vi "turn off a light.vi"(6 "error in":errorcluster, 7 "Which Button?":u32, 8 "Button 4":refnum<vi>, 9 "Button 3":refnum<vi>, 10 "Button 2":refnum<vi>, 11 "Button 1":refnum<vi>) -> (4 "error out":errorcluster)   [LabVIEW 2024]
panel:
  in  "Blank Button":bool
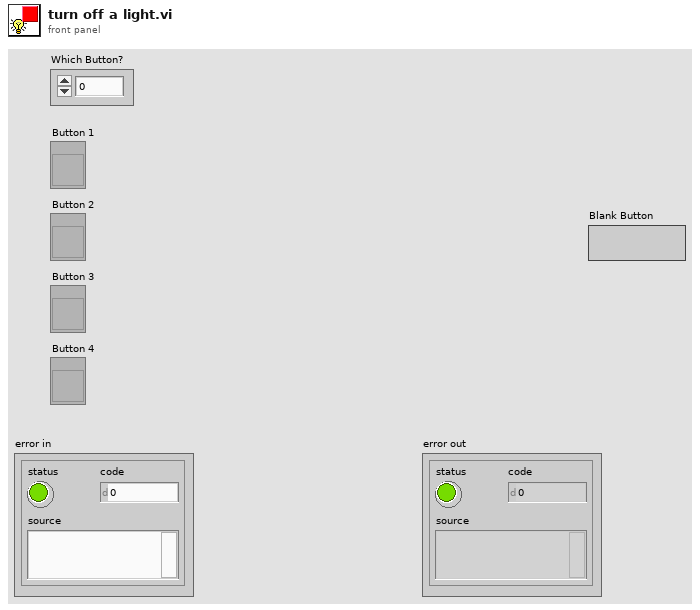
[diagram p1: front panel]
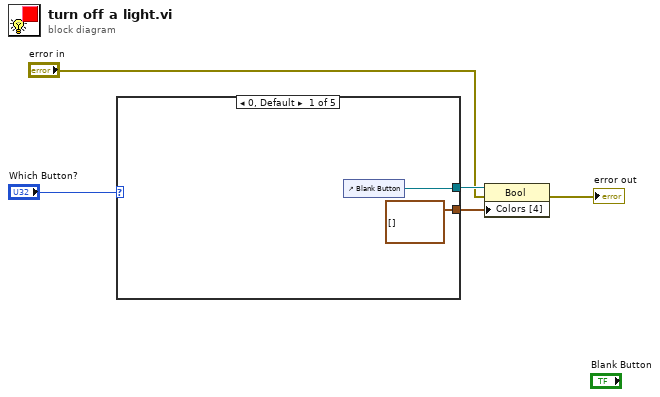
[diagram p0: block diagram]
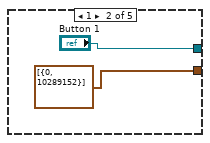
[diagram p2: hidden frame]
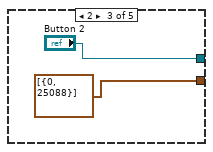
[diagram p3: hidden frame]
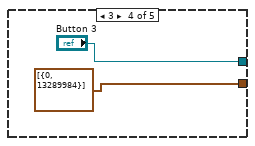
[diagram p4: hidden frame]
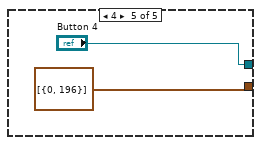
[diagram p5: hidden frame]
diagram:
  n1 = case shown="0, Default" "Which Button?" {
    tunnel: [w7 "Button 1" "Button 2" "Button 3" "Button 4"] -> w4
    tunnel: [cluster{u32, u32}[] [] ("Colors [4]") cluster{u32, u32}[] [{0, 10289152}] ("Colors [4]") cluster{u32, u32}[] [{0, 25088}] ("Colors [4]") cluster{u32, u32}[] [{0, 13289984}] ("Colors [4]") cluster{u32, u32}[] [{0, 196}] ("Colors [4]")] -> w3
    frame 0, Default {
      n2 = control-ref of="Blank Button"() -> (w7:refnum<vi>)
    }
    frame 1 {
    }
    frame 2 {
    }
    frame 3 {
    }
    frame 4 {
    }
  }
  n3 = property on="Property Node" class="Bool"(reference=w4, error in="error in", "Colors [4]"=w3) -> (error out=→"error out":errorcluster)  [unwired: 1 out]
